vi "Event handler-MovCor.vi"(10 "Movement Correction ON?":bool, 11 "UI queue in":refnum<queue>) -> (0 "error out":errorcluster)   [LabVIEW 2020]
uses:
  Queue/Message Queue/Typedefs/Message Cluster.ctl
  Typedefs/HW config states enum.ctl
  Typedefs/fgv_actions.ctl
  Global Variables/gl_UI Ctrl Refs.vi
  Global Variables/General Globals.vi
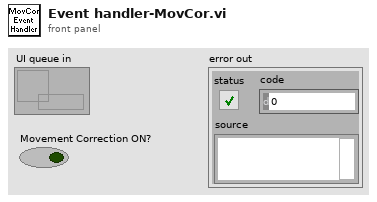
[diagram p1: front panel]
types:
  T1 = typedef "HW config states enum.ctl" = enum16{"Load from file", "Save to file", "Save backup", "Write all", "Read all", "Write XY stage settings", "Write DAQ FPGA settings", "Write Control FPGA settings", "Write Phys Channels", "Write System Config", "Write HW Config", "Save System Config", "Save HW Config", "Clear", "Compare from file"}
  T2 = typedef "Hardware Configuration settings.ctl" = cluster{"Dev. PC":bool, "Swap XY on stage":bool, "No of AOD":u8, "MC Supported":bool, "Axial MC":bool, "Computer MAC address":string, "Externalise Triggers":bool, "Trigger HW config":T3, "DAQmx Chan":T4, "XYZ Stage Control Config":T5, "XY stage available":bool, "XY Comms Config Cluster":T6, "Y stage available":bool, "Y Comms Config Cluster":T6, "Z stage available":bool, "Z Comms Config Cluster ":T6, "Encoder available":bool, "Encoder":T8, "VidRec available":bool, "Cam VidRec":T9, "Laser Power Control HW config":T10, "Laser 1 available":bool, "Laser 1 config cluster":T11, "Prechirper 1 available":bool, "Prechirper 1 config cluster":T12, "Control system.FPGA available?":bool, "Control Sys. HW config":T13, "DAQ FPGA HW Config":T14, "PMT Control Voltage Limits":T18}
  T3 = typedef "Triggers HW config.ctl" = cluster{"Available Device List":i32, "Device Address":string}
  T4 = typedef "DAQmx physical channels cluster.ctl" = cluster{"Pockels AO":tag, "Hard shutter AO":tag, "PMT AOs":tag, "Galvo AOs":tag, "Power meter AI":tag}
  T5 = typedef "XYZControlConfig.ctl" = enum16{"None", "XYZ", "XY-Z", "X-Y-Z", "Z"}
  T6 = typedef "Peripherals comms config cluster.ctl" = cluster{"Name":string, "Device Address":string, "Port ":u16, "Baudrate":i32, "Comms Type":T7}
  T7 = typedef "Comms Type.ctl" = enum16{"GPIB-IEEE488", "Serial-RS232", "Serial-RS485", "Serial-RS422", "Serial-USB", "Ethernet-TCP/IP", "Ethernet-UDP"}
  T8 = typedef "Encoder config cluster.ctl" = cluster{"IP address":string, "Port":u16, "Wheel radius (cm)":dbl, "Encoder Trigger":tag}
  T9 = typedef "Cam VidRec HW config setup cluster.ctl" = cluster{"DO flag-Video record":tag, "DO flag-Trial start":tag}
  T10 = typedef "Laser Power Control HW config.ctl" = cluster{"Laser Power Control":string, "Laser Power Modulation Control":enum16{"NI", "FPGA"}}
  T11 = typedef "Laser 1 config cluster.ctl" = cluster{"COM port":refnum<visa-resource-name>, "Baud Rate":i32, "Type":string}
  T12 = typedef "PreChirper 1 config cluster.ctl" = cluster{"Type":string, "Baud Rate":i32, "COM port":refnum<visa-resource-name>}
  T13 = typedef "Control Sys HW config cluster.ctl" = cluster{"Control system.FPGA Type":enum16{"Virtex 5", "Virtex 7"}, "Control system.Network adapter name":string, "Control system.MAC address":string, "Control system.Ethernet Port":u32, "Control system.Ethernet Port Opened":bool}
  T14 = typedef "DAQ FPGA HW config cluster.ctl" = cluster{"FGPA Ref":T15, "Target":T16, "input card type":T17}
  T15 = typedef "FPGA Ref.ctl" = refnum<k20>
  T16 = typedef "nirio_resource_hc.ctl" = tag
  T17 = typedef "FPGA input type AC-DC.ctl" = enum16{"AC Card", "DC Card"}
  T18 = typedef "PMT Control Voltage limits.ctl" = cluster{"Lower Limit":dbl, "Upper Limit":dbl}
  T19 = typedef "UI ctrl refs cluster.ctl" = cluster{"Top level VI path":path, "Top level VI ref":refnum<vi>, "User menu ref":refnum<k9>, "Sub Panel control":refnum<vi>, "Imaging Param Tab":refnum<vi>, "Occurrence-Start drivers":refnum<k4>, "Occurrence-Speed logging initialised":refnum<k4>, "Occurrence-XYZ stage initialised":refnum<k4>, "Exit button":refnum<vi>, "Status ind":refnum<vi>, "Set as origin":refnum<vi>, "Speed Logging":refnum<vi>, "Time Lapse":refnum<vi>, "Live Imaging":refnum<vi>, "AOL Z Stack":refnum<vi>, "Motor Z Stack":refnum<vi>, "Funct Acq button":refnum<vi>, "Hard Shutter":refnum<vi>, "Virtual Shutter":refnum<vi>, "Laser Power":refnum<vi>, "AOL Mode":refnum<vi>, "Frame Size":refnum<vi>, "Field of View":refnum<vi>, "Dwell Time":refnum<vi>, "Zoom":refnum<vi>, "AOL Z":refnum<vi>, "Objective":refnum<vi>, "Axis":refnum<vi>, "Paths & Names":refnum<vi>, "Experiment folder path (ind.)":refnum<vi>, "Last State (Ind.)":refnum<vi>, "Averages":refnum<vi>, "Angle (degrees)":refnum<vi>, "X centre":refnum<vi>, "Y centre":refnum<vi>, "Plane Mode":refnum<vi>, "# Planes":refnum<vi>, "Z Start":refnum<vi>, "Z Stop":refnum<vi>, "Z Step":refnum<vi>, "PMT 1":refnum<vi>, "PMT 2":refnum<vi>, "Stage XYZ Position":refnum<vi>, "Pockels@Z Start":refnum<vi>, "Pockels@Z Stop":refnum<vi>, "Obtain Z Start":refnum<vi>, "Obtain Z Stop":refnum<vi>, "Live stim.trig.period":refnum<vi>, "Live stim.trig.enable":refnum<vi>, "Movement Correction":refnum<vi>, "Load Reference Image":refnum<vi>, "XY Stage Move":refnum<vi>, "MovCor Cluster":refnum<vi>, "RefDAQParam":refnum<vi>, "Funct. Acq. Pockels Modulation":refnum<vi>, "Ref Laser Power":refnum<vi>, "Enable Video Recording":refnum<vi>, "Video Record-Live Imaging":refnum<vi>, "Video Record-Funct acq":refnum<vi>, "Reference Source":refnum<vi>, "AOL Z-stack Chirps Ready (ind)":refnum<vi>, "Target time between mov.cor. ref triggers (ms)":refnum<vi>, "Funct. Acq. Ref frame save":refnum<vi>, "Tracking button":refnum<vi>, "Show ref plots window":refnum<vi>, "Center freq ind (nm)":refnum<vi>, "Pickup mode (ind)":refnum<vi>, "Logging queue (ind)":refnum<vi>, "Back aperture power (ind.)":refnum<vi>, "Power after objective (ind.)":refnum<vi>, "Switch user":refnum<vi>, "Ls1 Conn. Status":refnum<vi>, "Ls1Tuning Status":refnum<vi>, "Ls1 Faults":refnum<vi>, "Ls1 Connection":refnum<vi>, "Ls1 Mode":refnum<vi>, "Ls1 POWER [mW]":refnum<vi>, "Ls1Shutter":refnum<vi>, "Ls1 Wavelength":refnum<vi>, "Ls1 Note":refnum<vi>, "Ls1 Confirm Wav":refnum<vi>, "Ls1 PreChrp Prism1":refnum<vi>, "Ls1 PreChrp Prism2":refnum<vi>, "Ls1 wav top Ind":refnum<vi>, "Ls1 power top Ind":refnum<vi>, "Ls1 Pump peak Hold":refnum<vi>, "Ls1 Status Ind":refnum<vi>, "Ls1 wav cancel":refnum<vi>, "Experiment Type":refnum<vi>, "Biology Information":refnum<vi>, "Camera recording status":refnum<vi>, "Optimise Obj. Pos.":refnum<vi>}
  T20 = enum8{"Enabled", "Disabled", "Disabled and Grayed Out"}
  T21 = typedef "fgv_actions.ctl" = enum16{"Get", "Set"}
  T22 = typedef "Reference_Globals.ctl" = cluster{"Refrence data path":path, "Reference Rectangle":i16[][], "AOL Z":dbl, "No of pixels in a miniscan ":i32[], "Threshold":i16[], "No of miniscans":i32[], "Full Frame Size":u16, "Reference Image":T23, "dwelltime":dbl, "Zoom":dbl, "Field of View":dbl, "Z Step":i8, "Z pixels":i32, "Z Lines":u8, "Z Ignore":u8, "Laser":u8, "Auto centering":bool}
  T23 = typedef "IMAQ Image.ctl" = refnum<image>
  T24 = typedef "AOL_Globals.ctl" = cluster{"Imaging Protocol":T25, "Number of POI":u16, "Number of Miniscans":u16, "Number of Trials":u16, "Number of Cycles ":u64, "# Averaged Frames":u16, "Laser power (%)":u8, "Pockels (V)":dbl, "Acquisition Length (sec)":dbl, "Fill time (us)":dbl, "POI Dwell time (us)":dbl, "Miniscan Dwell time per pixel (us)":dbl, "PMT 1":dbl, "PMT 2":dbl, "Back Apperture (mA)":dbl, "Frame Size":T26, "Center Frequency":dbl, "Field of View (um)":dbl, "Field of View (norm)":dbl, "DwellTime (us)":dbl, "Ref Dwell Time (us)":dbl, "Wavelength (nm)":dbl, "Zoom":dbl, "AOL Z":dbl, "AOL Mode":T27, "GridXY":dbl, "GridZ":dbl, "TriggerPeriod (sec)":dbl, "Number of Pixels in Miniscan":u16, "Experiment folder path":path, "X centre":dbl, "Y centre":dbl, "Angle (degrees)":dbl, "Angle Xs (degrees)":dbl, "Angle Ys (degrees)":dbl, "Plane Mode":T28, "Threshold":u16[], "Regenerate Chirps":bool, "Rectangle ROI length (pixels)":u16, "Rectangle ROI height (pixels)":u16, "AOD fill":u16, "StartupDelay":i32, "Samples Wait after Trigger":u16, "Slip Cycle":u32, "Add Cycle":bool, "Functional Mode":T29, "Z Start":dbl, "Z Stop":dbl, "# Planes":i32, "Total Pixels":i32, "Variable Miniscan Pixels":u16[], "Use Variable Length":bool, "Use Variable Resolution":bool, "Laser power (%) at Z Start":u8, "Laser power (%) at Z Stop":u8, "Ref Z Step":i8}
  T25 = typedef "Imaging Protocols enum.ctl" = enum16{"AOL Z-Stack", "Motor Z Stack", "Parameter Sweep", "Functional Acquisition", "Single Plane Acquisition", "Volume Acquisition", "Live Imaging", "Live Plane Imaging", "Live Volume Imaging"}
  T26 = typedef "Frame Size.ctl" = u16
  T27 = typedef "AOL modes.ctl" = enum16{"Raster", "Structural", "Pointing", "Mini Scan", "Alignment"}
  T28 = typedef "Plane Mode.ctl" = u16
  T29 = typedef "Functional Mode.ctl" = enum16{"Point", "Line", "Patch", "Plane", "Volume"}
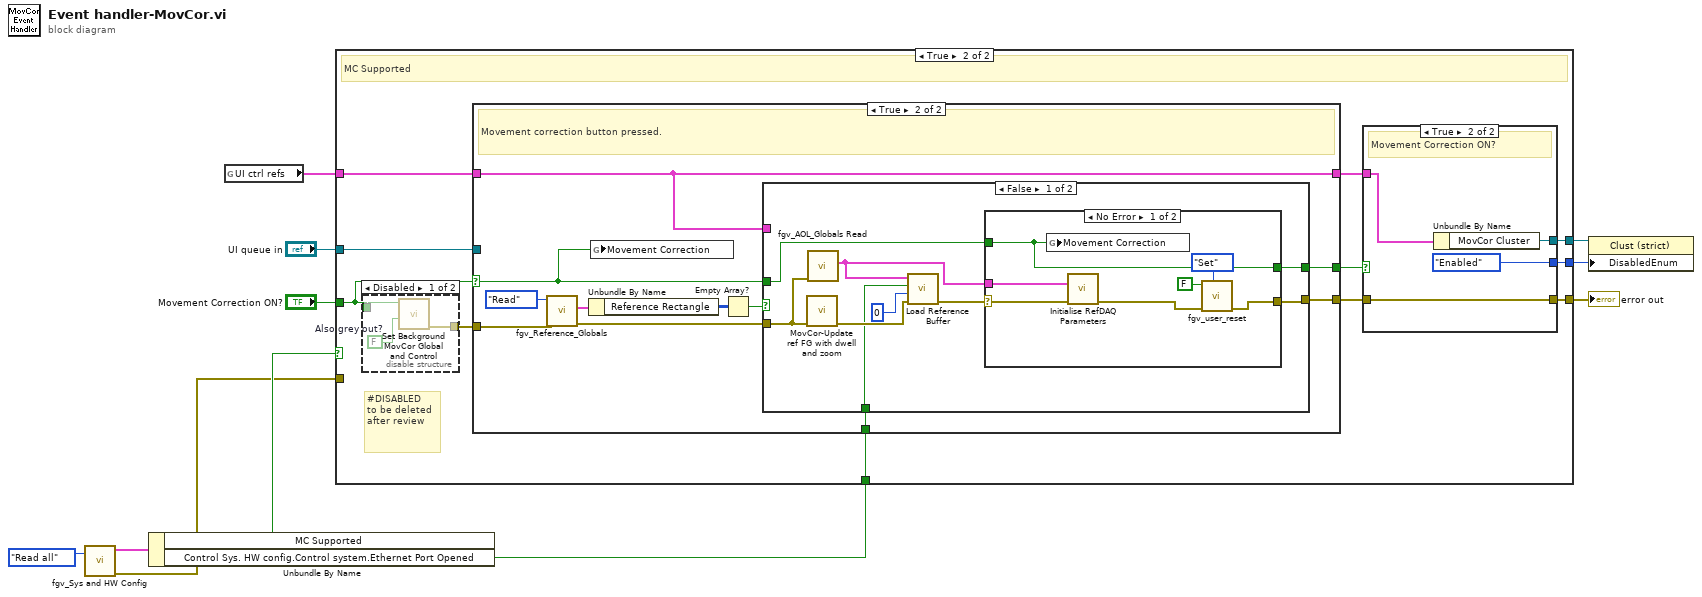
[diagram p0: block diagram]
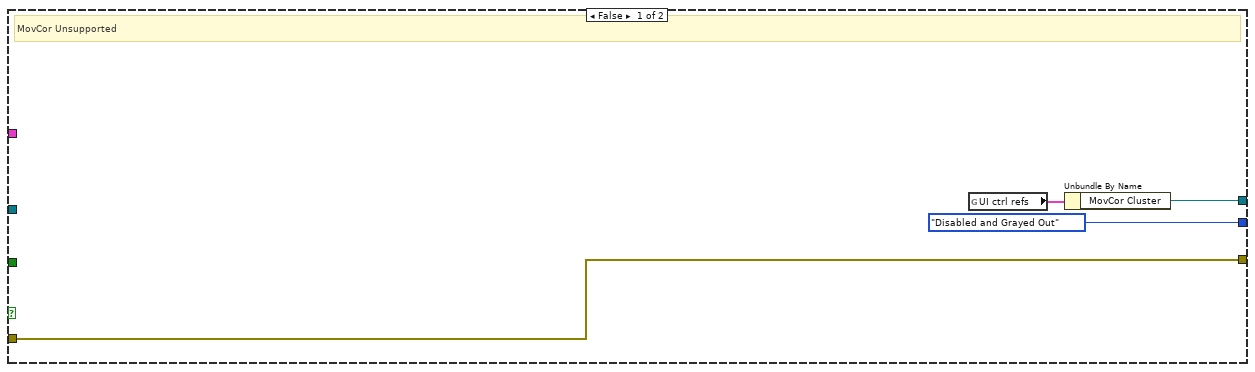
[diagram p2: hidden frame]
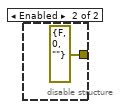
[diagram p3: hidden frame]
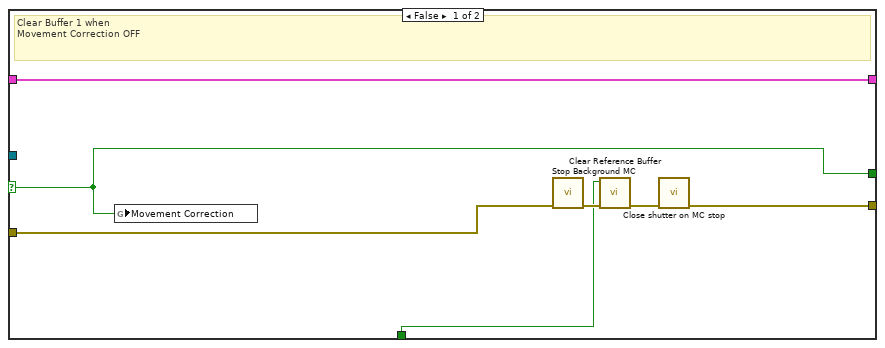
[diagram p4: hidden frame]
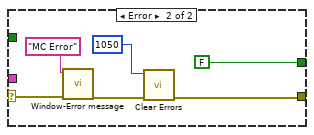
[diagram p5: hidden frame]
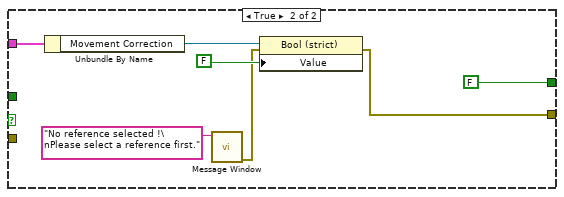
[diagram p6: hidden frame]
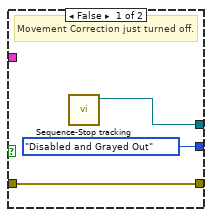
[diagram p7: hidden frame]
diagram:
  n1 = call "fgv_Sys and HW Config.vi"("Function"=HW_config_states_enum."Read all") -> ("error out"=w3:errorcluster, "Hardware Configuration OUT"=w7:T2)  [unwired: 8 in, 1 out]
  n2 = Unbundle By Name(w7) -> ("MC Supported"=w6:bool, "Control Sys. HW config.Control system.Ethernet Port Opened"=w1:bool)
  n3 = global read "gl_UI Ctrl Refs.vi" "UI ctrl refs"() -> (w2:T19)
  n4 = case shown="True" w6 {
    tunnel: [w14 w23] -> w11
    tunnel: "UI queue in" -> [_ w26]
    tunnel: "Movement Correction ON?" -> [_ w18]
    tunnel: [T20."Disabled and Grayed Out" ("Disabled") w22] -> w5
    tunnel: [w12 w21] -> w4
    tunnel: w3 -> [w14 _]
    tunnel: w2 -> [_ w20]
    tunnel: w1 -> [_ w17]
    frame False {
      # "MovCor Unsupported"
      n5 = global read "gl_UI Ctrl Refs.vi" "UI ctrl refs"() -> (w13:T19)
      n6 = Unbundle By Name(w13) -> ("MovCor Cluster"=w12:refnum<vi>)
    }
    frame True {
      # "#DISABLED\nto be deleted \nafter review"
      # "MC Supported"
      n7 = disable-structure shown="Disabled" {
        disable-tunnel: [w29 errorcluster {"status"=FALSE, "code"=0, "source"=""} ("error out")] -> w25
        disable-tunnel: w18 -> [w28 _]
        frame Disabled {
          w27 = FALSE  # Also grey out?
          n8 = call "Set Background MovCor Global and Control.vi"("Also grey out?"=w27, "On/Off"=w28) -> ("error out"=w29:errorcluster)  [unwired: 9 in]
        }
        frame Enabled {
        }
      }
      n9 = case shown="True" w18 {
        selector: w18 -> [w33 w38]
        tunnel: w26 -> [_ _]
        tunnel: [w31 w48] -> w24
        tunnel: w25 -> [w37 w42]
        tunnel: w20 -> [w35 w43]
        tunnel: [w35 w43] -> w19
        tunnel: w17 -> [w34 w40]
        tunnel: [w33 w39] -> w16
        frame False {
          # "Clear Buffer 1 when \nMovement Correction OFF"
          n10 = global write "General Globals.vi" "Movement Correction"(w33) -> ()
          n11 = call "Stop Background MC.vi"("error in (no error)"=w37) -> ("error out"=w36:errorcluster)  [unwired: 9 in, 1 out]
          n12 = call "Clear Reference Buffer.vi"("error in (no error)"=w36, "Ethernet port opened"=w34) -> ("error out"=w32:errorcluster)  [unwired: 9 in]
          n13 = call "Close shutter on MC stop.vi"("error in (no error)"=w32) -> ("error out"=w31:errorcluster)  [unwired: 10 in]
        }
        frame True {
          # "Movement correction button pressed."
          n14 = call "fgv_Reference_Globals.vi"("error in (no error)"=w42, "Function"=enum16{"Intialize", "Write", "Read", "Clear"}."Read") -> ("error out"=w41:errorcluster, "Reference Data"=w46:T22)  [unwired: 8 in]
          n15 = Unbundle By Name(w46) -> ("Reference Rectangle"=w45:i16[][])
          n16 = global write "General Globals.vi" "Movement Correction"(w38) -> ()
          n17 = Empty Array?(array=w45) -> (empty?=w44:bool)
          n18 = case shown="False" w44 {
            tunnel: [w55 w72] -> w48
            tunnel: w43 -> [_ w74]
            tunnel: w38 -> [w50 _]
            tunnel: w41 -> [w53 _]
            tunnel: w40 -> [w52 _]
            tunnel: [w49 FALSE] -> w39
            frame False {
              n19 = call "MovCor-Update ref FG with dwell and zoom.vi"("error in (no error)"=w53) -> ("error out"=w54:errorcluster)  [unwired: 10 in]
              n20 = call "fgv_AOL_Globals Read.vi"("error in (no error)"=w53) -> ("AOL_Globals"=w56:T24)  [unwired: 8 in, 2 out]
              n21 = call "Load Reference Buffer.vi"("error in (no error)"=w54, "Acquired z-plane index"=0, "Ethernet Port Opened ?"=w52, "AOL_Globals"=w56) -> ("error out"=w51:errorcluster)  [unwired: 7 in]
              n22 = case shown="No Error" w51 {
                selector: w51 -> [w63 w69]
                tunnel: w56 -> [w64 _]
                tunnel: [w58 w65] -> w55
                tunnel: w50 -> [w62 _]
                tunnel: [w62 FALSE] -> w49
                frame No Error {
                  n23 = global write "General Globals.vi" "Movement Correction"(w62) -> ()
                  n24 = call "Initialise RefDAQ Parameters.vi"("AOL Global"=w64, "error in (no error)"=w63) -> ("error out"=w59:errorcluster)  [unwired: 12 in, 1 out]
                  n25 = call "fgv_user_reset.vi"("FGV Actions"=fgv_actions."Set", "error in (no error)"=w59, "User reset"=FALSE) -> ("error out"=w58:errorcluster)  [unwired: 7 in, 1 out]
                }
                frame Error {
                  n26 = call "Window-Error message.vi"("error in (no error)"=w69, "Message"="MC Error") -> ("Error Out (no error)"=w66:errorcluster)  [unwired: 9 in]
                  n27 = call <vilib>:"Clear Errors.vi"("error in (no error)"=w66, "specific error code to clear (0: all)"=1050) -> ("error out"=w65:errorcluster)  [unwired: 4 in, 1 out]
                }
              }
            }
            frame True {
              n28 = Unbundle By Name(w74) -> ("Movement Correction"=w76:refnum<vi>)
              n29 = call "Message Window.vi"("Message string"="No reference selected !\nPlease select a reference first.") -> ("error out (no error)"=w73:errorcluster)  [unwired: 10 in]
              n30 = property class="Bool (strict)"(reference=w76, error in=w73, "Value"=FALSE) -> (error out=w72:errorcluster)  [unwired: 1 out]
            }
          }
        }
      }
      n31 = case shown="True" w16 {
        tunnel: w24 -> [w80 w84]
        tunnel: [w80 w84] -> w23
        tunnel: [T20."Disabled and Grayed Out" ("Disabled") T20."Enabled" ("Disabled")] -> w22
        tunnel: [w79 w82] -> w21
        tunnel: w19 -> [_ w81]
        frame False {
          # "Movement Correction just turned off."
          n32 = call "Sequence-Stop tracking.vi"() -> ("MovCor Cluster ref out"=w79:refnum<vi>)  [unwired: 11 in]
        }
        frame True {
          # "Movement Correction ON?"
          n33 = Unbundle By Name(w81) -> ("MovCor Cluster"=w82:refnum<vi>)
        }
      }
    }
  }
  "error out" <- w11
  n34 = property on="Property Node" class="Clust (strict)"(reference=w4, "DisabledEnum"=w5) -> ()  [unwired: 1 in, 2 out]
